vi "Update Gain Ranging FSM.vi"(0 "session in":T3[](array[typedef]) {"rx baseband session"."3630 session"."Address Space" items=["VXI/VME A16"=1, "VXI/VME A24"=2, "VXI/VME A32"=3, "VXI/VME A64"=4, "PXI Memory Allocations"=9, "PXI Configuration"=10, "PXI BAR0"=11, "PXI BAR1"=12, "PXI BAR2"=13, "PXI BAR3"=14, "PXI BAR4"=15, "PXI BAR5"=16]; "tx baseband session"."3610 session"."Address Space" items=["VXI/VME A16"=1, "VXI/VME A24"=2, "VXI/VME A32"=3, "VXI/VME A64"=4, "PXI Memory Allocations"=9, "PXI Configuration"=10, "PXI BAR0"=11, "PXI BAR1"=12, "PXI BAR2"=13, "PXI BAR3"=14, "PXI BAR4"=15, "PXI BAR5"=16]}, 1 "scope":string(combo), 5 "gain setting list":T1[](array[typedef]), 7 "gain dwell time (s)":dbl=2.5e-05 format="%#_6p", 11 "error in":errorcluster) -> (4 "session out":T3[](array[typedef]) {"rx baseband session"."3630 session"."Address Space" items=["VXI/VME A16"=1, "VXI/VME A24"=2, "VXI/VME A32"=3, "VXI/VME A64"=4, "PXI Memory Allocations"=9, "PXI Configuration"=10, "PXI BAR0"=11, "PXI BAR1"=12, "PXI BAR2"=13, "PXI BAR3"=14, "PXI BAR4"=15, "PXI BAR5"=16]; "tx baseband session"."3610 session"."Address Space" items=["VXI/VME A16"=1, "VXI/VME A24"=2, "VXI/VME A32"=3, "VXI/VME A64"=4, "PXI Memory Allocations"=9, "PXI Configuration"=10, "PXI BAR0"=11, "PXI BAR1"=12, "PXI BAR2"=13, "PXI BAR3"=14, "PXI BAR4"=15, "PXI BAR5"=16]}, 15 "error out":errorcluster)   [LabVIEW 2019]
uses:
  TypeDefs/Session.ctl
  <instrlib>/niMmWave/ni3620/Config/v1/Host/Public/High-Level/niMmWave Session.ctl
  <instrlib>/_niInstr/Register Bus/v0/Host/Public/Register Bus Session.ctl
  <instrlib>/_niInstr/Register Bus/v0/Host/Private/Session Data.ctl
  <instrlib>/niMmWave/ni3620/Config/v1/Host/Public/Typedefs/Board Information.ctl
  <instrlib>/niMmWave/ni3620/Config/v1/Host/Public/Typedefs/Hardware Revision.ctl
  <instrlib>/niMmWave/ni3620/Config/v1/Host/Public/Typedefs/Gain Mapping.ctl
  <instrlib>/niMmWave/ni3620/Config/v1/Host/Public/Typedefs/Correction Data.ctl
  <instrlib>/niMmWave/ni3620/Config/v1/Host/Public/Typedefs/Opera Characterization.ctl
  <instrlib>/niMmWave/ni3620/Config/v1/Host/Public/Corrections/Typedefs/Opera Characterization Main Header.ctl
  <instrlib>/niMmWave/ni3620/Config/v1/Host/Public/Corrections/Typedefs/Opera IF Board Information.ctl
  <instrlib>/niMmWave/ni3620/Config/v1/Host/Public/Corrections/Typedefs/Opera Characterization Instance Header.ctl
  <instrlib>/niMmWave/ni3620/Config/v1/Host/Public/Corrections/Typedefs/Opera Characterization Device Data Header.ctl
  <instrlib>/niMmWave/ni3620/Config/v1/Host/Public/Corrections/Typedefs/Opera LO Characterization Data Header.ctl
  <instrlib>/niMmWave/ni3620/Config/v1/Host/Public/Corrections/Typedefs/Opera IF Board Characterization Data Header.ctl
  <instrlib>/niMmWave/ni3620/Config/v1/Host/Public/Corrections/Typedefs/Opera Characterization Device Data.ctl
  <instrlib>/niMmWave/ni3620/Config/v1/Host/Public/Corrections/Typedefs/Opera LO2 Board Characterization Data.ctl
  <instrlib>/niMmWave/ni3620/Config/v1/Host/Public/Corrections/Typedefs/Opera LO Characterization Data.ctl
  <instrlib>/niMmWave/ni3620/Config/v1/Host/Public/Corrections/Typedefs/Opera IF Board Characterization Data.ctl
  <instrlib>/niMmWave/ni3620/Config/v1/Host/Public/Corrections/Typedefs/Opera IQ Impairment Data.ctl
  <instrlib>/niMmWave/ni3620/Config/v1/Host/Public/Typedefs/mmWave Adapter Session Data.ctl
  <instrlib>/niMmWave/ni3620/Config/v1/Host/Public/Typedefs/mmWave Adapter Data.ctl
  <instrlib>/niMmWave/ni3620/Config/v1/Host/Public/Typedefs/mmWave Adapter 2.ctl
  <instrlib>/niMmWave/ni3620/Config/v1/Shared/Typedefs/Subsystem ID.ctl
  <instrlib>/niMmWave/ni3620/Config/v1/Host/Public/Typedefs/mmWave Adapter Channel Information.ctl
  <instrlib>/niMmWave/ni3620/Config/v1/Host/Public/Typedefs/Temperature Coefficients.ctl
  <instrlib>/niMmWave/ni3620/Config/v1/Host/Public/Typedefs/mmWave Characterization.ctl
  <instrlib>/niMmWave/ni3620/Config/v1/Host/Public/Corrections/Typedefs/mmWave Characterization Main Header.ctl
  <instrlib>/niMmWave/ni3620/Config/v1/Host/Public/Corrections/Typedefs/mmWave Characterization Instance Header.ctl
  <instrlib>/niMmWave/ni3620/Config/v1/Host/Public/Typedefs/Session Cache.ctl
  <instrlib>/niMmWave/ni3620/Config/v1/Host/Public/Typedefs/LO2 settings cache.ctl
  <instrlib>/niMmWave/ni3620/Config/v1/Host/Public/Typedefs/LO2 source.ctl
  <instrlib>/niMmWave/ni3620/Config/v1/Host/Public/Typedefs/Desired and Coerced.ctl
  <instrlib>/niMmWave/ni3620/Config/v1/Host/Public/Typedefs/Export cache.ctl
  <instrlib>/niMmWave/ni3620/Config/v1/Host/Public/Typedefs/Path cache.ctl
  <instrlib>/niMmWave/ni3620/Config/v1/Host/Public/Typedefs/Daughterboard Type.ctl
  <instrlib>/niMmWave/ni3620/Config/v1/Host/Public/Typedefs/LO1 settings cache.ctl
  <instrlib>/niMmWave/ni3620/Config/v1/Host/Public/Typedefs/LO1 Source.ctl
  <instrlib>/niMmWave/ni3620/Config/v1/Host/Public/Typedefs/mmWave export cache.ctl
  <instrlib>/niMmWave/ni3620/Config/v1/Host/Private/Board/LO2/LO2 Board Configuration Cache.ctl
  <instrlib>/niMmWave/ni3620/Config/v1/Host/Public/Typedefs/reference clock routing settings.ctl
  <instrlib>/niMmWave/ni3620/Config/v1/Host/Public/Typedefs/LO2 routing settings.ctl
  <instrlib>/niMmWave/ni3620/Config/v1/Host/Private/Board/LO1/LO1 Board Configuration Cache.ctl
  <instrlib>/niMmWave/ni3620/Config/v1/Host/Public/Typedefs/LO1 source settings.ctl
  <instrlib>/niMmWave/ni3620/Config/v1/Host/Public/Typedefs/LO1 export settings.ctl
  <instrlib>/niMmWave/ni3620/Config/v1/Host/Public/Typedefs/LO1 mmWave settings.ctl
  TypeDefs/Tx Baseband Session.ctl
  <instrlib>/niMmWave/ni3610 and ni3630/controls/public/Main Settings.ctl
  <vilib>/Instr/_visa.llb/VISA Register Access Address Space.ctl
  <instrlib>/niMmWave/ni3610 and ni3630/controls/public/Register Adresses.ctl
  <instrlib>/niMmWave/ni3610 and ni3630/controls/public/Base Card Type.ctl
  <instrlib>/niMmWave/ni3610 and ni3630/controls/private/IQ Card Revision.ctl
  <instrlib>/niMmWave/ni3610 and ni3630/controls/public/Board Capability.ctl
  TypeDefs/Blank FPGA Reference.ctl
  TypeDefs/Rx Baseband Session.ctl
  TypeDefs/Hardware Configuration.ctl
  TypeDefs/Direction.ctl
  TypeDefs/Gain Ranging.ctl
  TypeDefs/PXI Trigger Bus Info.ctl
  TypeDefs/Gain Setting.ctl
  <instrlib>/niMmWave/ni3620/Config/v1/FPGA/Public/Typedefs/TX1 RX1 Port.ctl
  TypeDefs/Gain Ranging Reference.ctl
  <vilib>/rvi/errors/niLvFpgaAdjustHostInterfaceError.vi
  <vilib>/rvi/interface/nirviReadWriteControl/nirviReadWriteControl.xnode
  <vilib>/rvi/interface/Simulation/niFpgaSimulationCallBeginRW.vi
  NiFpgaLv.dll
  <instrlib>/_niInstr/Register Bus/v0/Host/niInstr Register Bus v0 Host.lvlib
  <instrlib>/niMmWave/ni3620/Config/v1/Host/niMmWave Config v1 Host.lvlib
  <instrlib>/niMmWave/ni3610 and ni3630/ni3610_and_ni3630_Driver_Lib.lvlib
  <instrlib>/niMmWave/ni3620/Config/v1/Shared/niMmWave Config v1 Shared.lvlib
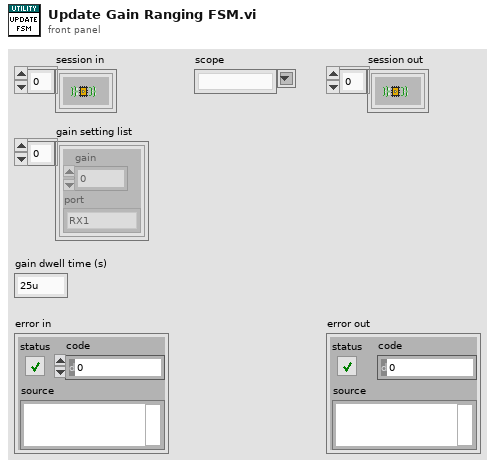
[diagram p1: front panel]
types:
  T1 = typedef "Gain Setting.ctl" = cluster{"gain":fxp<+/-,16,12>, "port":T2}
  T2 = typedef "TX1 RX1 Port.ctl" = enum8{"RX1", "TX1/RX2"}
  T3 = typedef "Session.ctl" = cluster{"3620 session":refnum<queue>, "tx baseband session":T4, "rx baseband session":T12, "tx gain (dB)":dbl, "rx gain (dB)":dbl, "hardware configuration":T13, "gain ranging":T15[], "pxi trigger bus information":T16}
  T4 = typedef "Tx Baseband Session.ctl" = cluster{"3610 session":T5, "7902 reference":T11}
  T5 = typedef "ni3610_and_ni3630_Driver_Lib.lvlib/Main Settings.ctl" = cluster{"VISA resource name":refnum<visa-resource-name>, "Address Space":T6, "window_offset":u32, "register_addresses":T7, "required_MM_fpga_version":cluster{"signature":u32, "hardware":u32, "current revision":u32, "oldest revision":u32}, "CPLD Oldest Compat Version ":cluster{"hardware":u32, "CPLD firmware":u32}, "MM_FPGA_image_location":string, "is_init":bool, "card_type":T8, "DacLmkConfigFileName":string, "AdcLmkConfigFileName":string, "AdcConfigFileName":string, "DacConfigFileName_RevA":string, "DacConfigFileName_RevB":string, "Mulde hardware revision":u8, "bypass DAC PLL\n":bool, "IQ Card Revision":T9, "board capability":T10}
  T6 = typedef "VISA Register Access Address Space.ctl" = u16
  T7 = typedef "ni3610_and_ni3630_Driver_Lib.lvlib/Register Adresses.ctl" = cluster{"MM based Registers":cluster{"Revision":u32, "OldestCompatRev":u32, "signature":u32, "scratch":u32, "LedControl":u32, "BoardHwRev":u32, "BoardControl":u32, "ThermalStatus":u32, "BasebandStatus":u32, "BasebandControl":u32, "BasebandAuxSetup":u32, "BasebandAuxStatus":u32, "LmkSyncOutSetup":u32, " AdcSyncOutSetup":u32, " InjSyncOutSetup":u32, " PxiTrig0OutSetup":u32, " PxiTrig1OutSetup":u32, " PxiTrig2OutSetup":u32, " PxiTrig3OutSetup":u32, " PxiTrig4OutSetup":u32, " PxiTrig5OutSetup":u32, " PxiTrig6OutSetup":u32, " PxiTrig7OutSetup":u32}, "CPLD based Registers":cluster{"SlaveSignature":u32, "SlaveRevision":u32, "SlaveOldestCompatRev":u32, "SlaveScratch":u32, "SlaveSetup":u32, "SlaveStatus":u32, "IDacReg_offset":u32, "LMKRegGrp0_offset":u32, "QDacReg_offset":u32, "BrdTempSensorVal":u32, "TempSensorPowerDown":u32, "GPIOReg_offset":u32, "IAdcReg_offset":u32, "QAdcReg_offset":u32, "LMKRegGrp1_offset":u32, "QadcTempSensorVal":u32, "IadcTempSensorVal":u32, "RevisionReg":u32, "VcxoReg":u32, "CpldStatusReg":u32, "PowerReg":u32, "VBiasEnReg":u32, "ExtRefOeReg":u32, "QdacCtrlReg":u32, "QdacStatusReg":u32, "IdacCtrlReg":u32, "IdacStatusReg":u32, "QdacJtagIn":u32, "QdacJtagOut":u32, "IdacJtagIn":u32, "IdacJtagOut":u32, "IqDcSetupReg":u32, "QadcStatusReg":u32, "IadcStatusReg":u32, "BrdSetupReg":u32, "IqDcRevisionReg":u32, "PllStatusReg":u32, "EndpointScratchReg":u32, "AdcSyncCfgReg":u32, "IqCardOpampReg":u32}, "CPLD Register Offset":u32, "MM  Register Offset":u32, " PxiTrig0OutSetup":u32}
  T8 = typedef "ni3610_and_ni3630_Driver_Lib.lvlib/Base Card Type.ctl" = enum16{"unspecified", "ADC", "DAC"}
  T9 = typedef "ni3610_and_ni3630_Driver_Lib.lvlib/IQ Card Revision.ctl" = enum16{"RevA", "RevB", "RevC", "RevD"}
  T10 = typedef "ni3610_and_ni3630_Driver_Lib.lvlib/Board Capability.ctl" = cluster{"baseband sync":enum16{"no baseband sync", "baseband sync"}}
  T11 = typedef "Blank FPGA Reference.ctl" = refnum<k20>
  T12 = typedef "Rx Baseband Session.ctl" = cluster{"3630 session":T5, "7902 reference":T11}
  T13 = typedef "Hardware Configuration.ctl" = cluster{"direction":T14, "baseband only":bool}
  T14 = typedef "Direction.ctl" = enum16{"Transceiver", "Receiver", "Transmitter"}
  T15 = typedef "Gain Ranging.ctl" = cluster{"gain ranging active scope":string, "gain ranging stream session":refnum<k20>}
  T16 = typedef "PXI Trigger Bus Info.ctl" = cluster{"chassis resource name":refnum<visa-resource-name>, "7902R (TX)":i16, "3610 (TX)":i16, "3620 (IF)":i16, "3630 (RX)":i16, "7902R (RX)":i16}
  T17 = cluster{"setting list write address":u32, "data":cluster{"gain":fxp<+/-,16,12>, "port":enum8{"RX1", "TX1/RX2"}}, "setting list size":u16}
  T18 = typedef "Gain Ranging Reference.ctl" = refnum<k20>
  T19 = typedef "Constants.ctl" = cluster{"data clock rate (Hz)":dbl, "sample rate (Hz)":dbl, "sample rate selector string":string, "default tx bitfile path":path, "default rx bitfile path":path, "default proc bitfile path":path}
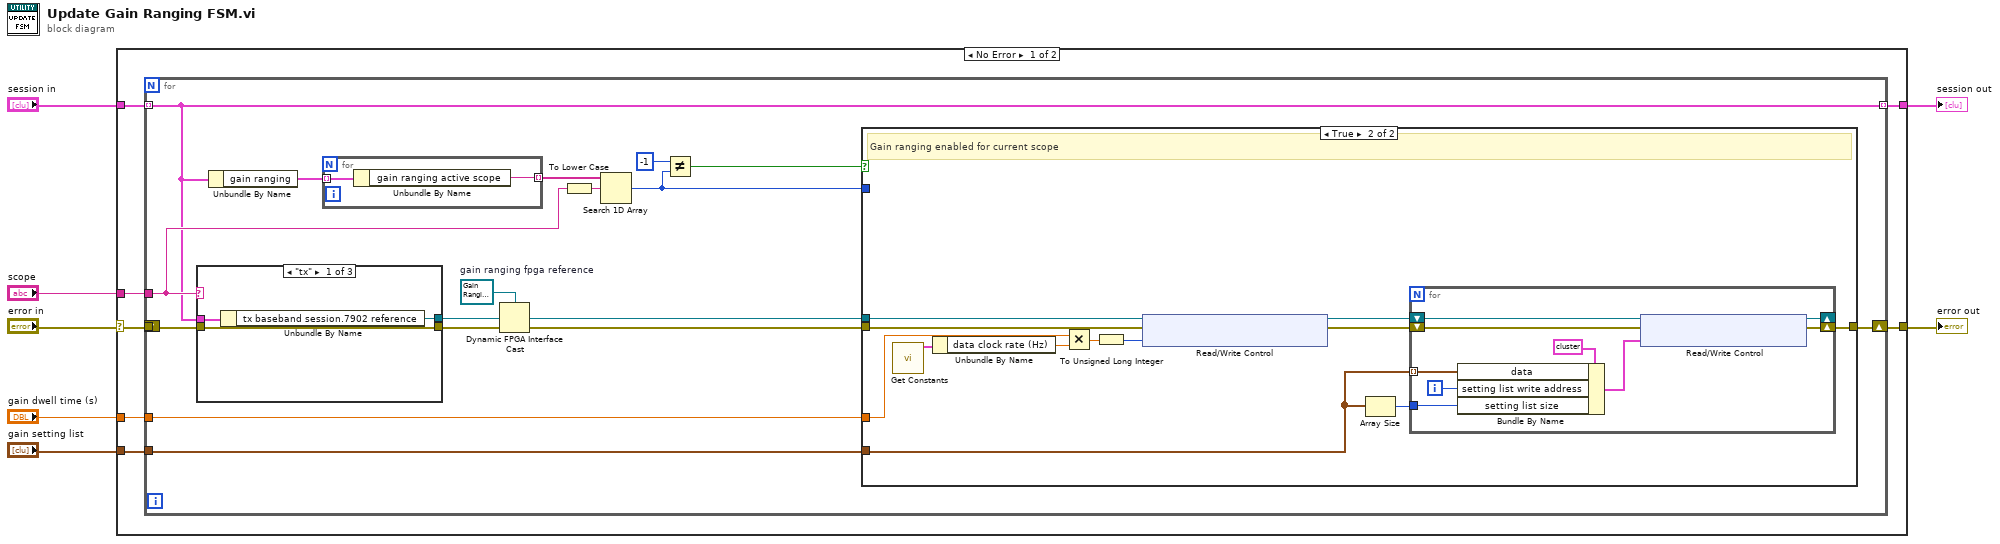
[diagram p0: block diagram]
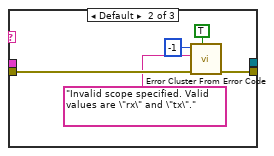
[diagram p2: hidden frame]
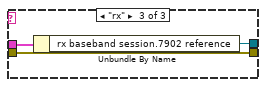
[diagram p3: hidden frame]
diagram:
  n1 = case shown="No Error" "error in" {
    selector: "error in" -> [w9 w67]
    tunnel: [w14 w67] -> w7
    tunnel: "session in" -> [w13 w66]
    tunnel: "scope" -> [w11 _]
    tunnel: "gain dwell time (s)" -> [w12 _]
    tunnel: [w10 w66] -> w3
    tunnel: "gain setting list" -> [w8 _]
    frame No Error {
      n2 = for {
        shift-right: [w29] -> w14
        shift-left: w9 -> [w24]
        tunnel: w13 -> [w15] mode=indexing
        tunnel: w12 -> [w26]
        tunnel: w8 -> [w25]
        tunnel: w11 -> [w18]
        tunnel: [w15] -> w10 mode=indexing
        tunnel: w9 -> [_]
        w28 = T18 refnum  # gain ranging fpga reference
        n3 = case shown="\"tx\"" w18 {
          tunnel: [w33 w39 w43] -> w16
          tunnel: w24 -> [w33 w40 w43]
          tunnel: w15 -> [w35 _ w42]
          tunnel: [w34 _ w41] -> w27
          frame "tx" {
            n4 = Unbundle By Name(w35) -> ("tx baseband session.7902 reference"=w34:T11)
          }
          frame Default {
            n5 = call <vilib>:"Error Cluster From Error Code.vi"("show call chain? (False)"=TRUE, "error in (no error)"=w40, "error message (\"\")"="Invalid scope specified. Valid values are \"rx\" and \"tx\"." ("error message (\"\")"), "error code (0)"=-1) -> ("error out"=w39:errorcluster)  [unwired: 5 in]
          }
          frame "rx" {
            n6 = Unbundle By Name(w42) -> ("rx baseband session.7902 reference"=w41:T11)
          }
        }
        n7 = Unbundle By Name(w15) -> ("gain ranging"=w21:T15[])
        n8 = for {
          tunnel: w21 -> [w32] mode=indexing
          tunnel: [w31] -> w23 mode=indexing
          n9 = Unbundle By Name(w32) -> ("gain ranging active scope"=w31:string)
        }
        n10 = Dynamic FPGA Interface Cast(Session In=w28, Type=w27) -> (Session Out=w30:T18)
        n11 = To Lower Case(string=w18) -> (all lower case string=w22:string)
        n12 = Search 1D Array(1D array=w23, element=w22) -> (index of element=w19:i32)  [unwired: 1 in]
        n13 = Not Equal?(x=-1, y=w19) -> (x != y?=w17:bool)
        n14 = case shown="True" w17 {
          tunnel: w30 -> [_ w56]
          tunnel: [w44 w45] -> w29
          tunnel: w16 -> [w44 w55]
          tunnel: w26 -> [_ w54]
          tunnel: w25 -> [_ w53]
          tunnel: w19 -> [_ _]
          frame False {
            # "Gain ranging disabled for current scope. Do nothing"
          }
          frame True {
            # "Gain ranging enabled for current scope"
            n15 = call "Get Constants.vi"() -> ("constants"=w47:T19)  [unwired: 15 in]
            n16 = Unbundle By Name(w47) -> ("data clock rate (Hz)"=w46:dbl)
            n17 = Multiply(x=w54, y=w46) -> (x*y=w52:dbl)
            n18 = To Unsigned Long Integer(number=w52) -> (unsigned 32bit integer=w51:u32)
            n19 = xnode "Read/Write Control"("FPGA VI Reference In"=w56, "error in"=w55, "gain ranging.dwell time (cycles)"=w51) -> ("FPGA VI Reference Out"=w48:T18, "error out"=w49:errorcluster)
            n20 = Array Size(array=w53) -> (size(s)=w50:i32)
            n21 = for {
              shift-right: [w65] -> w45
              shift-left: w49 -> [w63]
              tunnel: w53 -> [w62] mode=indexing
              shift-right: [w64] -> _
              shift-left: w48 -> [w60]
              tunnel: w50 -> [w59]
              i -> [w61]
              n22 = Bundle By Name(cluster=T17 {"setting list write address"=0, "data"={"gain"=0.0, "port"=enum."RX1"}, "setting list size"=0} ("gain ranging.setting list step"), "data"=w62, "setting list write address"=w61, "setting list size"=w59) -> (w57:T17)
              n23 = xnode "Read/Write Control"("FPGA VI Reference In"=w60, "error in"=w63, "gain ranging.setting list step"=w57) -> ("FPGA VI Reference Out"=w64:T18, "error out"=w65:errorcluster)
            }
          }
        }
      }
    }
    frame Error {
    }
  }
  "error out" <- w7
  "session out" <- w3
